vi "Read TimeRefType.vi"(8 "error in (no error)":errorcluster, 11 "NiPxi6683H in":refnum<class "NiPxi6683H.lvclass">) -> (0 "error out":errorcluster, 2 "TimeRefType":T1=enum."GPS", 3 "NiPxi6683H out":refnum<class "NiPxi6683H.lvclass">)   [LabVIEW 2014, in "SyncPlugins.lvlib" / "NiPxi6683H.lvclass"]
uses:
  NiPxi6683H.lvclass
  PXI_MultiTrig/Typedefs/TimeRefType.ctl
  NiPxi6683H.lvclass/NiPxi6683H.ctl
  PXI_MultiTrig/PXI_MultiTrig.lvclass
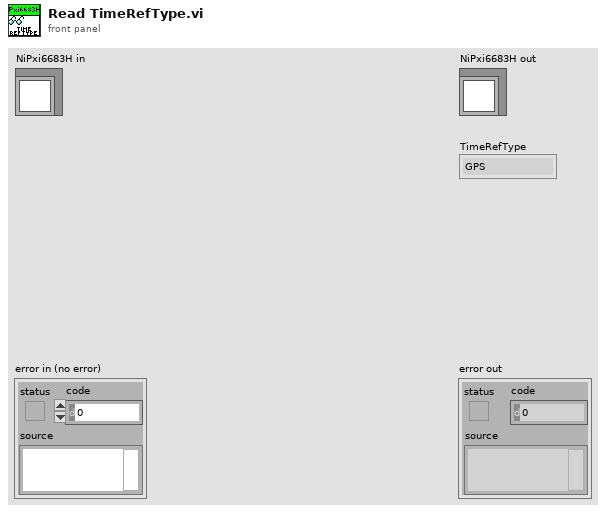
[diagram p1: front panel]
types:
  T1 = typedef "SyncPlugins.lvlib/PXI_MultiTrig.lvclass/TimeRefType.ctl" = enum16{"1588", "Free Running", "GPS", "IRIG", "PPS"}
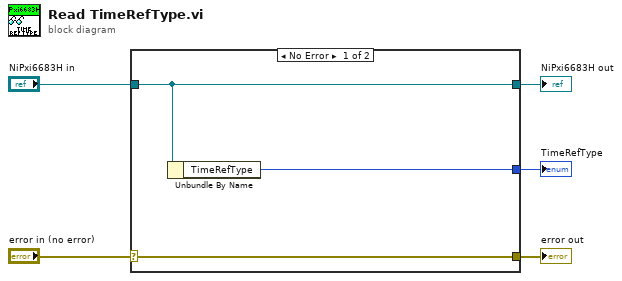
[diagram p0: block diagram]
diagram:
  n1 = case shown="No Error" "error in (no error)" {
    selector: "error in (no error)" -> [w8 w9]
    tunnel: [w8 w9] -> w4
    tunnel: [w7 w10] -> w2
    tunnel: "NiPxi6683H in" -> [w7 w10]
    tunnel: [w6 _] -> w1
    frame No Error {
      n2 = Unbundle By Name(w7) -> ("TimeRefType"=w6:T1)
    }
    frame Error {
    }
  }
  "error out" <- w4
  "NiPxi6683H out" <- w2
  "TimeRefType" <- w1
